vi "LNLS Control PS Data to LOCON_BIPOLAR_16BITS Data.vi"(8 "error in (no error)":errorcluster, 9 "PS Status (On correction?)":bool[](array[boolean]), 10 "PS Status (ON/OFF)":bool[](array[boolean]), 11 "PS Readings/Setpoints":dbl[](array[numeric])) -> (0 "error out":errorcluster, 3 "PS Readings/Setpoints LOCON Data":T1[](array[typedef]) {"status" format="%08b"})   [LabVIEW 2011, in "LNLS Control VIs.lvlib"]
uses:
  LNLS Control VIs.lvlib
  Types Definitions/Type LOCON_BIPOLAR_16BITS.ctl
  Type Definitions.lvlib
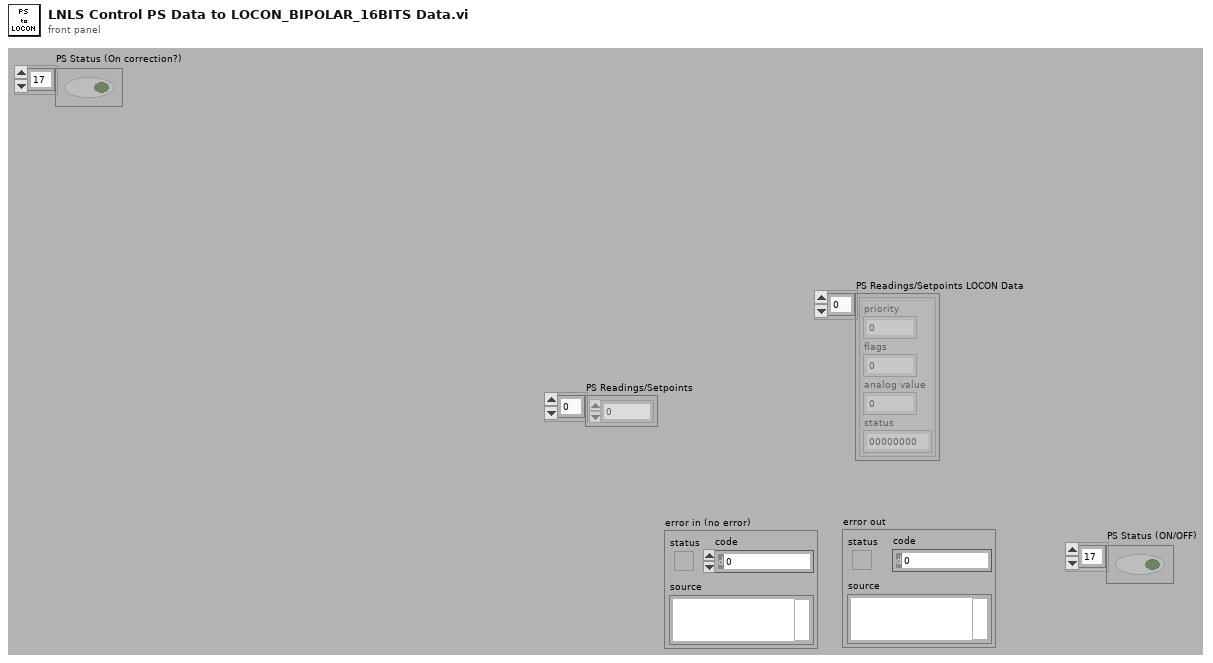
[diagram p1: front panel]
types:
  T1 = typedef "Type Definitions.lvlib/Type LOCON_BIPOLAR_16BITS.ctl" = cluster{"priority":u8, "flags":u8, "analog value":u16, "status":u8}
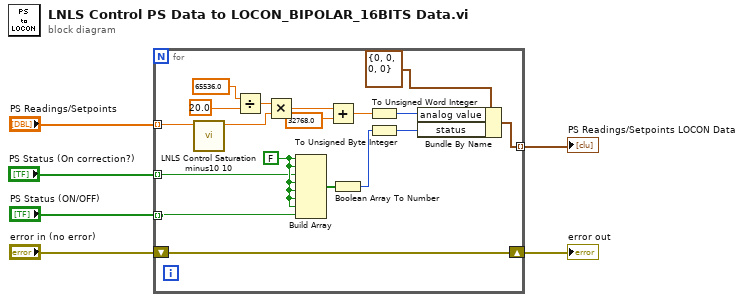
[diagram p0: block diagram]
diagram:
  n1 = for {
    tunnel: [w24] -> w3 mode=indexing
    shift-right: [w19] -> w5
    shift-left: "error in (no error)" -> [w19]
    tunnel: "PS Readings/Setpoints" -> [w12] mode=indexing
    tunnel: "PS Status (ON/OFF)" -> [w16] mode=indexing
    tunnel: "PS Status (On correction?)" -> [w13] mode=indexing
    w14 = FALSE ("element")
    n2 = call "LNLS Control Saturation minus10 10.vi"("in"=w12) -> ("saturated out"=w11:dbl)  [unwired: 10 in]
    n3 = Divide(x=65536.0, y=20.0) -> (x/y=w18:dbl)
    n4 = Multiply(x=w18, y=w11) -> (x*y=w21:dbl)
    n5 = Build Array(w14, w14, w13, w14, w14, w14, w14, w16) -> (w15:bool[])
    n6 = Add(x=w21, y=32768.0) -> (x+y=w10:dbl)
    n7 = Boolean Array To Number(Boolean array=w15) -> (number=w8:u32)
    n8 = To Unsigned Word Integer(number=w10) -> (unsigned 16bit integer=w9:u16)
    n9 = To Unsigned Byte Integer(number=w8) -> (unsigned 8bit integer=w7:u8)
    n10 = Bundle By Name(cluster=T1 {"priority"=0, "flags"=0, "analog value"=0, "status"=0}, "analog value"=w9, "status"=w7) -> (w24:T1)
  }
  "PS Readings/Setpoints LOCON Data" <- w3
  "error out" <- w5
